vi "PARTICLE_DETECT.vi"(0 "Range (Threshold 1)":cluster{"Lower value":sgl, "Upper value":sgl}={"Lower value"=128.0, "Upper value"=255.0}, 1 "Min Radius (Circle Detection 1)":sgl=5.0, 7 "error in":errorcluster, 8 "File Path":path=path "C:/SNAPSHOT.bmp") -> (20 "Nb Circles (Circle Detection 1)":i32=3, 21 "Circles Data (Circle Detection 1)":T2(array[cluster]), 27 "error out":errorcluster)   [LabVIEW 2014]
uses:
  <vilib>/vision/NI_Vision_Development_Module.lvlib
panel:
  out "Image Out":T1(plugin-control)
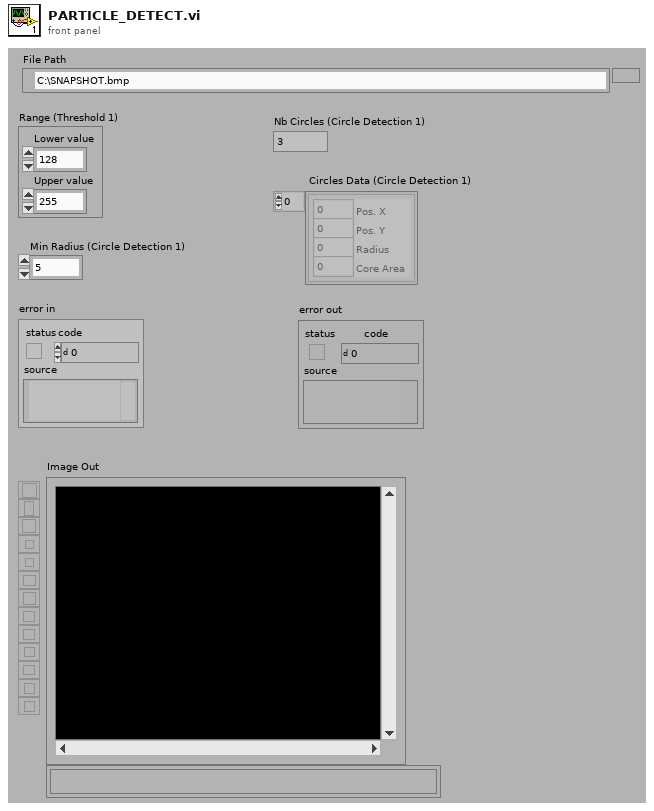
[diagram p1: front panel]
types:
  T1 = typedef "IMAQ Image.ctl" = refnum<image>
  T2 = cluster{"Pos. X":i32, "Pos. Y":i32, "Radius":i32, "Core Area":i32}[]
  T3 = typedef "Image Type" = u32
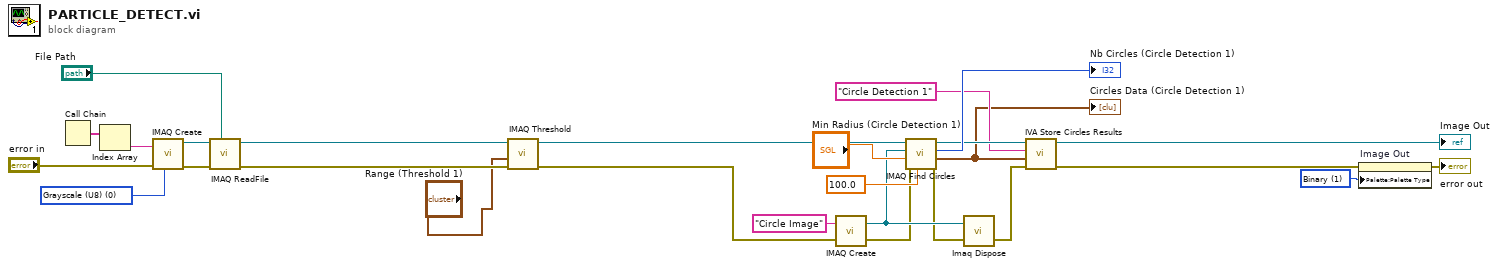
[diagram p0: block diagram]
diagram:
  w3 = u32 1 items=["Grayscale", "Binary", "Gradient", "Rainbow", "Temperature", "User Defined"] ("Palette")
  w20 = T3 0 items=["Grayscale (U8)", "Grayscale (I16)", "Grayscale (SGL)", "Complex (CSG)", "RGB (U32)", "HSL (U32)", "RGB (U64)", "Grayscale (U16)"] ("Image Type")
  n1 = Call Chain() -> (call chain=w22:string[])
  n2 = Index Array(array=w22) -> (element=w21:string)  [unwired: 1 in]
  n3 = call "IMAQ Create"("Image Name"=w21, "Image Type"=w20, "error in (no error)"="error in") -> ("New Image"=w25:T1, "error out"=w24:errorcluster)  [unwired: 1 in, 1 out]
  n4 = call "IMAQ ReadFile"("File Path"="File Path", "error in (no error)"=w24, "Image"=w25) -> ("error out"=w26:errorcluster, "Image Out"=w18:T1)  [unwired: 2 in, 5 out]
  n5 = call "IMAQ Threshold"("error in (no error)"=w26, "Range"="Range (Threshold 1)", "Image Src"=w18) -> ("error out"=w17:errorcluster, "Image Dst Out"=w7:T1)  [unwired: 3 in, 4 out]
  n6 = call "IMAQ Create"("Image Name"="Circle Image", "error in (no error)"=w17) -> ("New Image"=w12:T1, "error out"=w11:errorcluster)  [unwired: 2 in, 1 out]
  n7 = call "IMAQ Find Circles"("Max Radius"=sgl 100.0, "error in (no error)"=w11, "Min Radius"="Min Radius (Circle Detection 1)", "Image Dst"=w12, "Image Src"=w7) -> ("error out"=w10:errorcluster, "Circles Data"=w5:T2, "Nb Circles"=→"Nb Circles (Circle Detection 1)":i32)  [unwired: 4 out]
  "Circles Data (Circle Detection 1)" <- w5
  n8 = call "Imaq Dispose"("Image"=w12, "error in (no error)"=w10) -> ("error out"=w9:errorcluster)  [unwired: 1 in, 3 out]
  n9 = call <vilib>:"IVA Store Circles Results.vi"("error in (no error)"=w9, "Circles Data"=w5, "Step Name"="Circle Detection 1", "Image in"=w7) -> ("error out"=w8:errorcluster, "Image dup"=→"Image Out":T1)  [unwired: 6 out]
  n10 = property on="Image Out" class="ImageControl"(error in=w8, "Palette:Palette Type"=w3) -> (error out=→"error out":errorcluster)  [unwired: 1 in, 1 out]
